vi "Create - Periodic Signal.vi"(0 "reference in":refnum<class "GSwFormDSP.lvclass">, 5 "error in (no error)":errorcluster) -> (14 "reference in":refnum<class "GSwFormDSP.lvclass">, 19 "error out":errorcluster)   [LabVIEW 2022 SP3, in "GSwFormDSP.lvclass"]
uses:
  GSwFormDSP.lvclass
  <vilib>/Analysis/NI_AALBase.lvlib
panel:
  in  "Phase (Deg)":dbl min=0.0 max=360.0 step=1.0 format="%.2f"
  in  "Signal Type":T1(ring)
  out "FS":dbl
  in  "Done":bool
  in  "Duration (s)":dbl=10.0 min=1.0 max=3600.0 step=0.1 format="%.1f"
  in  "User Input Fs":T2(ring)=enum."44100 Hz" caption="Sampling Rate"
  in  "Frequency (Hz)":dbl=1000.0 min=0.0 max=22050.0 step=1.0 format="%.2f"
  in  "Amplitude":dbl=1.0 format="%.2f"
  in  "Signal Name":string="unknown"
  in  "Signal Unit":string="unknown"
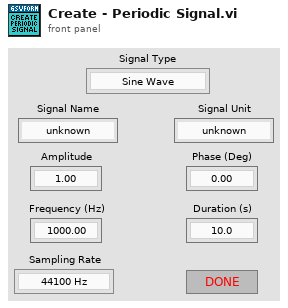
[diagram p1: front panel]
types:
  T1 = enum16{"Sine Wave", "Triangle Wave", "Square Wave", "Sawtooth Wave"}
  T2 = enum16{"256 Hz", "512 Hz", "1024 Hz", "2048 Hz", "4096 Hz", "8192 Hz", "11025 Hz", "16384 Hz", "22050 Hz", "32768 Hz", "44100 Hz"}
  T3 = enum16{"Replace Current Signals", "Append to Current Signals"}
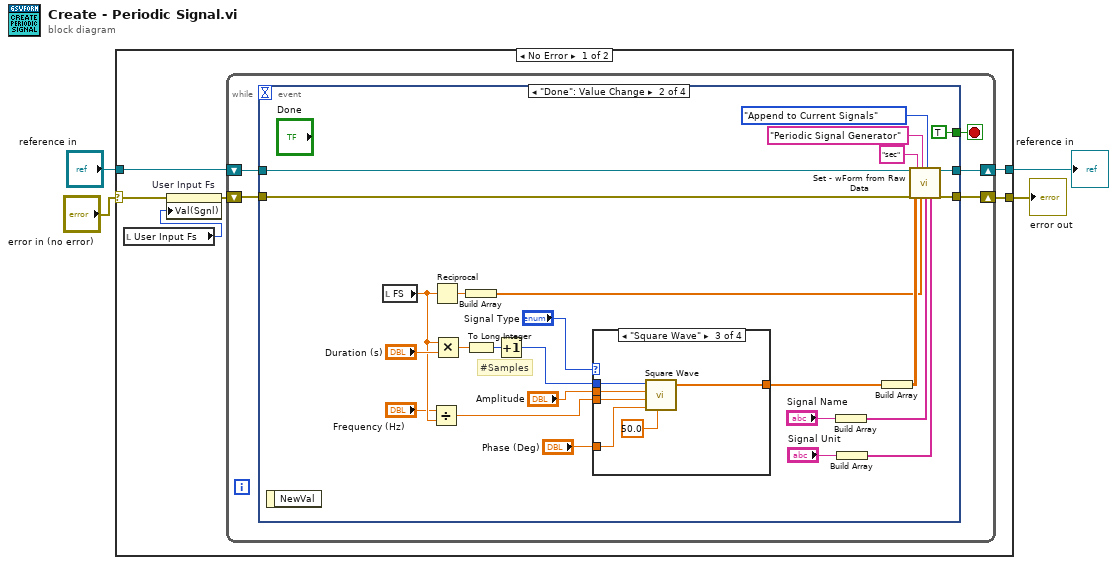
[diagram p0: block diagram]
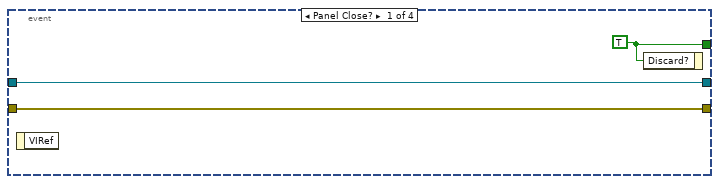
[diagram p2: hidden frame]
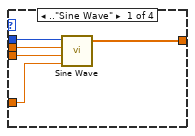
[diagram p3: hidden frame]
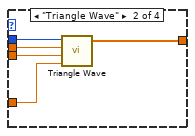
[diagram p4: hidden frame]
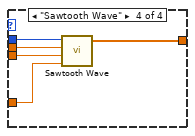
[diagram p5: hidden frame]
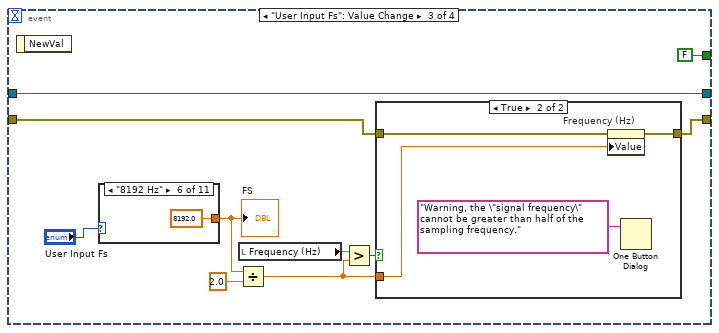
[diagram p6: hidden frame]
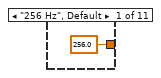
[diagram p8: hidden frame]
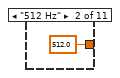
[diagram p9: hidden frame]
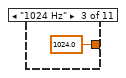
[diagram p10: hidden frame]
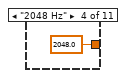
[diagram p11: hidden frame]
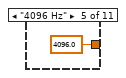
[diagram p12: hidden frame]
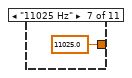
[diagram p13: hidden frame]
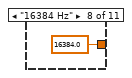
[diagram p14: hidden frame]
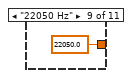
[diagram p15: hidden frame]
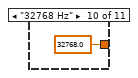
[diagram p16: hidden frame]
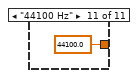
[diagram p17: hidden frame]
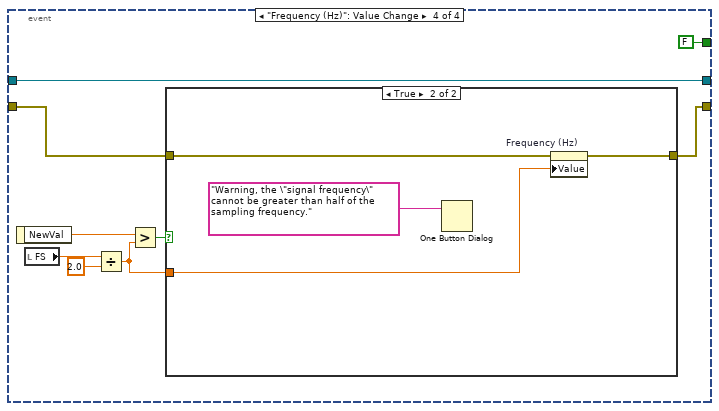
[diagram p18: hidden frame]
diagram:
  n1 = case shown="No Error" "error in (no error)" {
    selector: "error in (no error)" -> [w5 w107]
    tunnel: [w8 w107] -> w3
    tunnel: [w9 w106] -> w1
    tunnel: "reference in" -> [w10 w106]
    frame No Error {
      n2 = local read "User Input Fs"() -> (w6:T2)
      n3 = property on="User Input Fs" class="Enum (strict)"(error in=w5, "Val(Sgnl)"=w6) -> (error out=w7:errorcluster)  [unwired: 1 in, 1 out]
      n4 = while {
        shift-right: [w13] -> w9
        shift-left: w10 -> [w14]
        shift-right: [w12] -> w8
        shift-left: w7 -> [w11]
        stop <- w15 stop-if-true
        n5 = event shown="[1] \"Done\": Value Change" {
          selector: _ -> [_ _ _ _]
          dyn-events: _ -> [_ _ _ _]
          timeout: _ -> [_ _ _ _]
          tunnel: [w18 TRUE ("Discard?") FALSE ("Discard?") FALSE ("Discard?")] -> w15
          tunnel: w14 -> [w17 w31 w73 w99]
          tunnel: [w17 w30 w73 w99] -> w13
          tunnel: [w16 w29 w67 w95] -> w12
          tunnel: w11 -> [w16 w28 w68 w96]
          event Panel Close? {
            w18 = TRUE ("Discard?")
            n6 = event-data() -> ()  [unwired: 1 in, 1 out]
            n7 = event-data("Discard?"=w18) -> ()  [unwired: 1 in, 1 out]
          }
          event "Done": Value Change {
            # "#Samples"
            n8 = event-data() -> ()  [unwired: 1 in, 1 out]
            n9 = local read "FS"() -> (w20:dbl)
            n10 = Divide(x="Frequency (Hz)", y=w20) -> (x/y=w21:dbl)
            n11 = Reciprocal(x=w20) -> (1/x=w41:dbl)
            n12 = Multiply(x=w20, y="Duration (s)") -> (x*y=w43:dbl)
            n13 = Build Array(w41) -> (w37:dbl[])
            n14 = To Long Integer(number=w43) -> (32bit integer=w42:i32)
            n15 = Increment(x=w42) -> (x+1=w25:i32)
            n16 = case shown="\"Square Wave\"" "Signal Type" {
              tunnel: w21 -> [w49 w54 w60 w65]
              tunnel: "Amplitude" -> [w48 w53 w59 w64]
              tunnel: w25 -> [w47 w52 w58 w63]
              tunnel: "Phase (Deg)" -> [w46 w51 w57 w62]
              tunnel: [w45 w50 w56 w61] -> w26
              frame .."Sine Wave" {
                n17 = call <vilib>:"Sine Wave.vi"("samples"=w47, "amplitude"=w48, "frequency"=w49, "phase in"=w46) -> ("sine wave"=w45:dbl[])  [unwired: 1 in, 2 out]
              }
              frame "Triangle Wave" {
                n18 = call <vilib>:"Triangle Wave.vi"("samples"=w52, "amplitude"=w53, "frequency"=w54, "phase in"=w51) -> ("triangle wave"=w50:dbl[])  [unwired: 1 in, 2 out]
              }
              frame "Square Wave" {
                n19 = call <vilib>:"Square Wave.vi"("samples"=w58, "amplitude"=w59, "frequency"=w60, "duty cycle (%)"=50.0, "phase in"=w57) -> ("square wave"=w56:dbl[])  [unwired: 1 in, 2 out]
              }
              frame "Sawtooth Wave" {
                n20 = call <vilib>:"Sawtooth Wave.vi"("samples"=w63, "amplitude"=w64, "frequency"=w65, "phase in"=w62) -> ("sawtooth wave"=w61:dbl[])  [unwired: 1 in, 2 out]
              }
            }
            n21 = Build Array("Signal Name") -> (w36:string[])
            n22 = Build Array("Signal Unit") -> (w35:string[])
            n23 = Build Array(w26) -> (w38:dbl[][])
            n24 = call "Set - wForm from Raw Data.vi"("reference in"=w31, "error in (no error)"=w28, "X Unit"="sec", "Y Data (Row matrix)"=w38, "Data Origin"="Periodic Signal Generator", "dTs"=w37, "Signal Set"=T3."Append to Current Signals", "Signals Name"=w36, "Signals Unit"=w35) -> ("reference in"=w30:refnum<class "GSwFormDSP.lvclass">, "error out"=w29:errorcluster)  [unwired: 9 in]
          }
          event "User Input Fs": Value Change {
            n25 = event-data() -> ()  [unwired: 1 in, 1 out]
            n26 = case shown="\"8192 Hz\"" "User Input Fs" {
              tunnel: [256.0 512.0 1024.0 2048.0 4096.0 8192.0 11025.0 16384.0 22050.0 32768.0 44100.0] -> w71
              frame "256 Hz", Default {
              }
              frame "512 Hz" {
              }
              frame "1024 Hz" {
              }
              frame "2048 Hz" {
              }
              frame "4096 Hz" {
              }
              frame "8192 Hz" {
              }
              frame "11025 Hz" {
              }
              frame "16384 Hz" {
              }
              frame "22050 Hz" {
              }
              frame "32768 Hz" {
              }
              frame "44100 Hz" {
              }
            }
            "FS" <- w71
            n27 = Divide(x=w71, y=2.0) -> (x/y=w66:dbl)
            n28 = local read "Frequency (Hz)"() -> (w70:dbl)
            n29 = Greater?(x=w70, y=w66) -> (0:w69:bool)
            n30 = case shown="True" w69 {
              tunnel: w68 -> [w76 w78]
              tunnel: [w76 w77] -> w67
              tunnel: w66 -> [_ w79]
              frame False {
              }
              frame True {
                n31 = property on="Frequency (Hz)" class="DigNum (strict)"(error in=w78, "Value"=w79) -> (error out=w77:errorcluster)  [unwired: 1 in, 1 out]
                n32 = One Button Dialog(message="Warning, the \"signal frequency\" cannot be greater than half of the sampling frequency.") -> ()  [unwired: 1 in, 1 out]
              }
            }
          }
          event "Frequency (Hz)": Value Change {
            n33 = event-data() -> ("NewVal"=w97:dbl)  [unwired: 1 in]
            n34 = local read "FS"() -> (w93:dbl)
            n35 = Divide(x=w93, y=2.0) -> (x/y=w92:dbl)
            n36 = Greater?(x=w97, y=w92) -> (0:w98:bool)
            n37 = case shown="True" w98 {
              tunnel: w96 -> [w101 w104]
              tunnel: [w101 w103] -> w95
              tunnel: w92 -> [_ w102]
              frame False {
              }
              frame True {
                n38 = One Button Dialog(message="Warning, the \"signal frequency\" cannot be greater than half of the sampling frequency.") -> ()  [unwired: 1 in, 1 out]
                n39 = property on="Frequency (Hz)" class="DigNum (strict)"(error in=w104, "Value"=w102) -> (error out=w103:errorcluster)  [unwired: 1 in, 1 out]
              }
            }
          }
        }
      }
    }
    frame Error {
    }
  }
  "error out" <- w3
  "reference in" <- w1
